vi "Turret.vi"   [LabVIEW 2012]
uses:
  StateMachineEnum.ctl
  Robot Global Data.vi
types:
  T1 = typedef "StateMachineEnum.ctl" = enum16{"Init", "Idle", "Start", "Do", "Stop"}
  T2 = typedef "WPI_MotorControlDeviceRef.ctl" = cluster{"DeviceStatus":errorcluster, "Type":enum16{"PWM", "CAN"}, "PWM":cluster{"Digital Module":T3, "PWM Channel":T4, "DeadBand":T5}, "CAN":cluster{"Device Number":u8, "Control Mode":T6, "Semaphore":T7, "Max Vout":dbl}, "Invert":bool, "TransformRef":T8, "InvTransformRef":T8}
  T3 = typedef "FPGA_TypedefDigitalModule.ctl" = enum16{"Digital Module 1", "Digital Module 2"}
  T4 = typedef "FPGA_DIOPWMChannel.ctl" = enum8{"PWM 1", "PWM 2", "PWM 3", "PWM 4", "PWM 5", "PWM 6", "PWM 7", "PWM 8", "PWM 9", "PWM 10", "Invalid"}
  T5 = typedef "WPI_PWMDeadband.ctl" = cluster{"Name":string, "maxPositivePwm":i32, "minPositivePwm":i32, "centerPwm":i32, "maxNegativePwm":i32, "minNegativePwm":i32, "angularRange":u16}
  T6 = typedef "WPI_CANJaguar_ControlMode.ctl" = enum8{"Percent VBus", "Current", "Speed", "Position", "Voltage"}
  T7 = typedef "Semaphore RefNum" = refnum<k1>
  T8 = typedef "WPI_PWMTransform_ConPane.ctl" = refnum<vi>
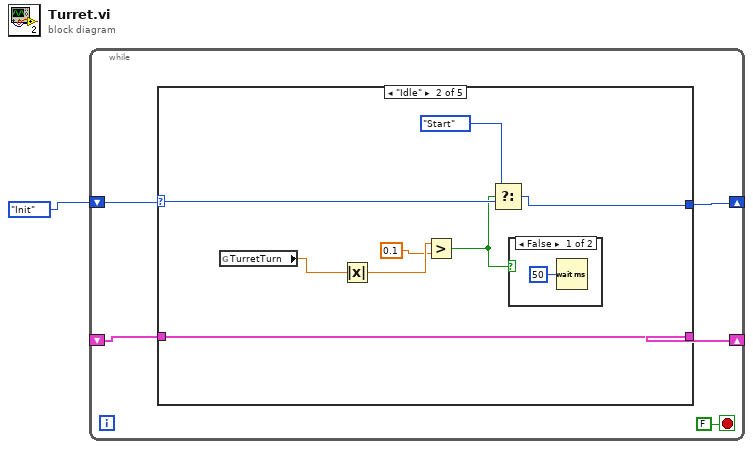
[diagram p0: block diagram]
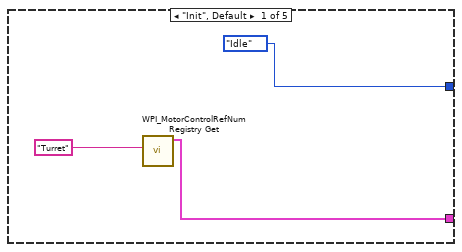
[diagram p2: hidden frame]
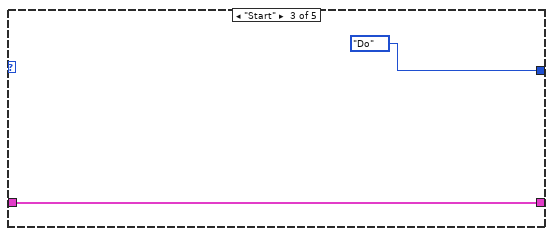
[diagram p4: hidden frame]
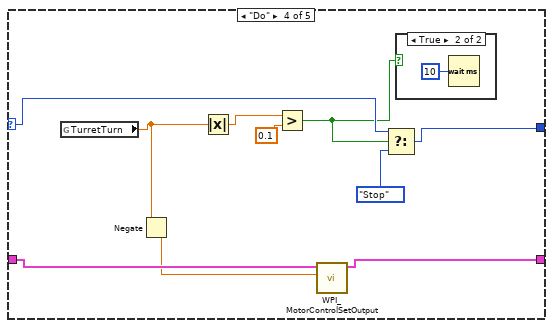
[diagram p5: hidden frame]
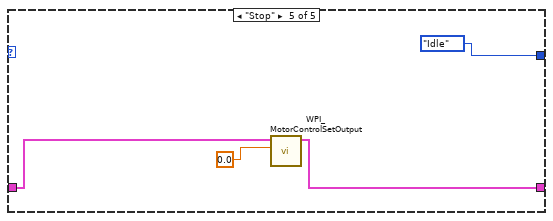
[diagram p7: hidden frame]
diagram:
  n1 = while {
    shift-right: [w6] -> _
    shift-left: _ -> [w3]
    shift-right: [w4] -> _
    shift-left: StateMachineEnum."Init" ("State") -> [w5]
    stop <- FALSE stop-if-true
    n2 = case shown="\"Idle\"" w5 {
      selector: w5 -> [_ w16 _ w24 _]
      tunnel: [w7 w17 w20 w29 w34] -> w6
      tunnel: [StateMachineEnum."Idle" ("State") w12 StateMachineEnum."Do" ("State") w25 StateMachineEnum."Idle" ("State")] -> w4
      tunnel: w3 -> [_ w17 w20 w30 w35]
      frame "Init", Default {
        n3 = call <vilib>:"WPI_MotorControlRefNum Registry Get.vi"("refnum name"="Turret") -> ("MotorControlDevRef"=w7:T2)  [unwired: 9 in, 1 out]
      }
      frame "Idle" {
        n4 = global read "Robot Global Data.vi" "TurretTurn"() -> (w11:dbl)
        n5 = Absolute Value(x=w11) -> (abs(x)=w15:dbl)
        n6 = Greater?(x=w15, y=0.1) -> (0:w10:bool)
        n7 = Select(t=StateMachineEnum."Start" ("State"), s=w10, f=w16) -> (s? t:f=w12:T1)
        n8 = case shown="False" w10 {
          frame False {
            n9 = Wait (ms)(milliseconds to wait=u32 50) -> ()  [unwired: 1 out]
          }
          frame True {
          }
        }
      }
      frame "Start" {
      }
      frame "Do" {
        n10 = global read "Robot Global Data.vi" "TurretTurn"() -> (w22:dbl)
        n11 = Negate(x=w22) -> (-x=w21:dbl)
        n12 = Absolute Value(x=w22) -> (abs(x)=w27:dbl)
        n13 = Greater?(x=w27, y=0.1) -> (0:w23:bool)
        n14 = call <vilib>:"WPI_MotorControlSetOutput.vi"("Output"=w21, "MotorControlDevRef"=w30) -> ("MotorControlDevRef"=w29:T2)  [unwired: 7 in, 2 out]
        n15 = Select(t=w24, s=w23, f=StateMachineEnum."Stop" ("State")) -> (s? t:f=w25:T1)
        n16 = case shown="True" w23 {
          frame False {
          }
          frame True {
            n17 = Wait (ms)(milliseconds to wait=u32 10) -> ()  [unwired: 1 out]
          }
        }
      }
      frame "Stop" {
        n18 = call <vilib>:"WPI_MotorControlSetOutput.vi"("Output"=0.0, "MotorControlDevRef"=w35) -> ("MotorControlDevRef"=w34:T2)  [unwired: 7 in, 2 out]
      }
    }
  }
